vi "Refnum To Path.vi"(6 "error in":errorcluster, 9 "Refnum":refnum<file>) -> (1 "UTF-8 Path":refnum<class "UTF-8 Path.lvclass">, 4 "error out":errorcluster)   [LabVIEW 2020, in "G-Unicode.lvlib"]
doc: "Returns the <b>UTF-8 Path</b> associated with the specified <b>Refnum</b>."
uses:
  G-Unicode.lvlib
  Types/UTF-8 Path/UTF-8 Path.lvclass
  Types/UTF-8 String/UTF-8 String.lvclass/UTF-8 String.ctl
  Types/UTF-8 Path/UTF-8 Path.lvclass/UTF-8 Path.ctl
  Short Name to Path.vi/f844562b-b612-4fa1-b092-3cf87b2107aa.vi
  Types/UTF-8 Path/Write Encoded UTF-8 Path.vi
  Types/UTF-8 String/Read Encoded UTF-8 String.vi
  Types/UTF-8 String/Write Encoded UTF-8 String.vi
  Private/Conversion/Text as Encoded String.vi
  Private/Conversion/Polymorphic VIs/Text as Encoded String (LabVIEW Path).vi
  Unicode/Encoded UTF-8 String to Encoded UTF-16LE String.vi
  Unicode/Encoded UTF-16LE String to Encoded UTF-8 String.vi
  Types/UTF-8 String/UTF-8 String.lvclass
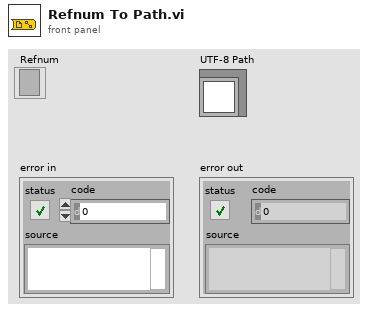
[diagram p1: front panel]
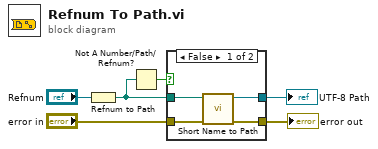
[diagram p0: block diagram]
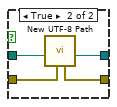
[diagram p2: hidden frame]
diagram:
  n1 = Refnum to Path(1:"Refnum") -> (0:w2:path)
  n2 = Not A Number/Path/Refnum?(number/path/refnum=w2) -> (NaN/Path/Refnum?=w1:bool)
  n3 = case shown="False" w1 {
    tunnel: w2 -> [w10 w14]
    tunnel: "error in" -> [w9 w13]
    tunnel: [w7 w12] -> w4
    tunnel: [w8 w11] -> w3
    frame False {
      n4 = call "Short Name to Path.vi"("error in"=w9, "LabVIEW Path"=w10) -> ("error out"=w7:errorcluster, "UTF-8 Path"=w8:refnum<class "UTF-8 Path.lvclass">)  [unwired: 8 in]
    }
    frame True {
      n5 = call "New UTF-8 Path.vi"("error in"=w13, "LabVIEW Path"=w14) -> ("UTF-8 Path"=w11:refnum<class "UTF-8 Path.lvclass">, "error out"=w12:errorcluster)  [unwired: 8 in]
    }
  }
  "UTF-8 Path" <- w3
  "error out" <- w4
